vi "user info.vi"(7 "枚举":enum16{"open", "write", "read", "close"}(ring), 8 "error in":errorcluster caption="错误输出", 9 "测试条件 in":T2, 10 "粉尘特性 in":T1, 11 "Test Information in":cluster{"Test Name":string, "Tester":string}) -> (0 "error out":errorcluster, 1 "测试条件":T2, 2 "粉尘特性":T1, 3 "Test Information":cluster{"Test Name":string, "Tester":string})   [LabVIEW 2011]
uses:
  <vilib>/Utility/config.llb/Write Key (String).vi
  <vilib>/Utility/config.llb/Write Key (Double).vi
  <vilib>/Utility/config.llb/Read Key (String).vi
  <vilib>/Utility/config.llb/Read Key (Double).vi
  <vilib>/Utility/config.llb/NI_LVConfig.lvlib
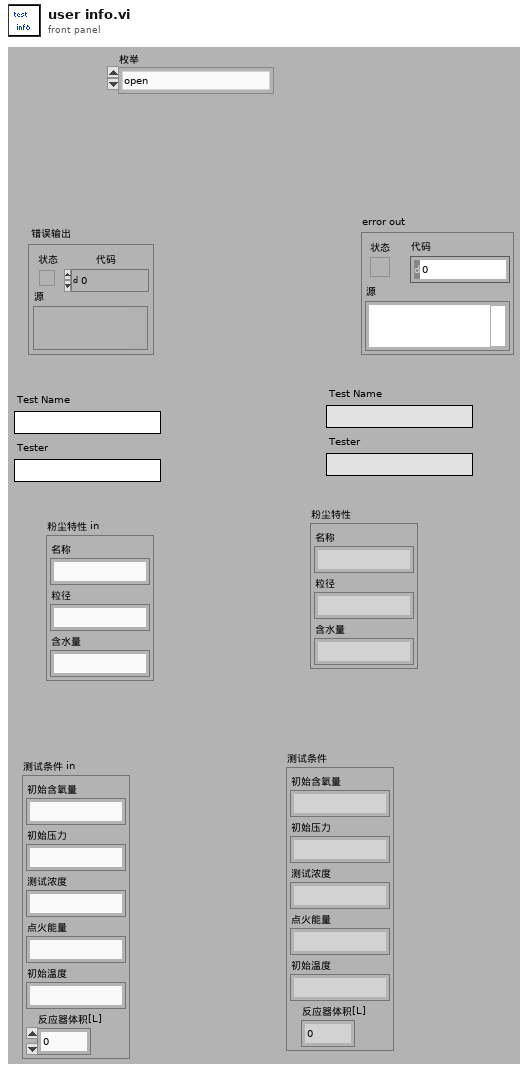
[diagram p1: front panel]
types:
  T1 = typedef "粉尘特性.ctl" = cluster{"名称":string, "粒径":string, "含水量":string}
  T2 = typedef "测试条件.ctl" = cluster{"初始含氧量":string, "初始压力":string, "测试浓度":string, "点火能量":string, "初始温度":string, "反应器体积[L]":dbl}
  T3 = typedef "NI_LVConfig.lvlib/Config Data RefNum.ctl" = refnum<k1>
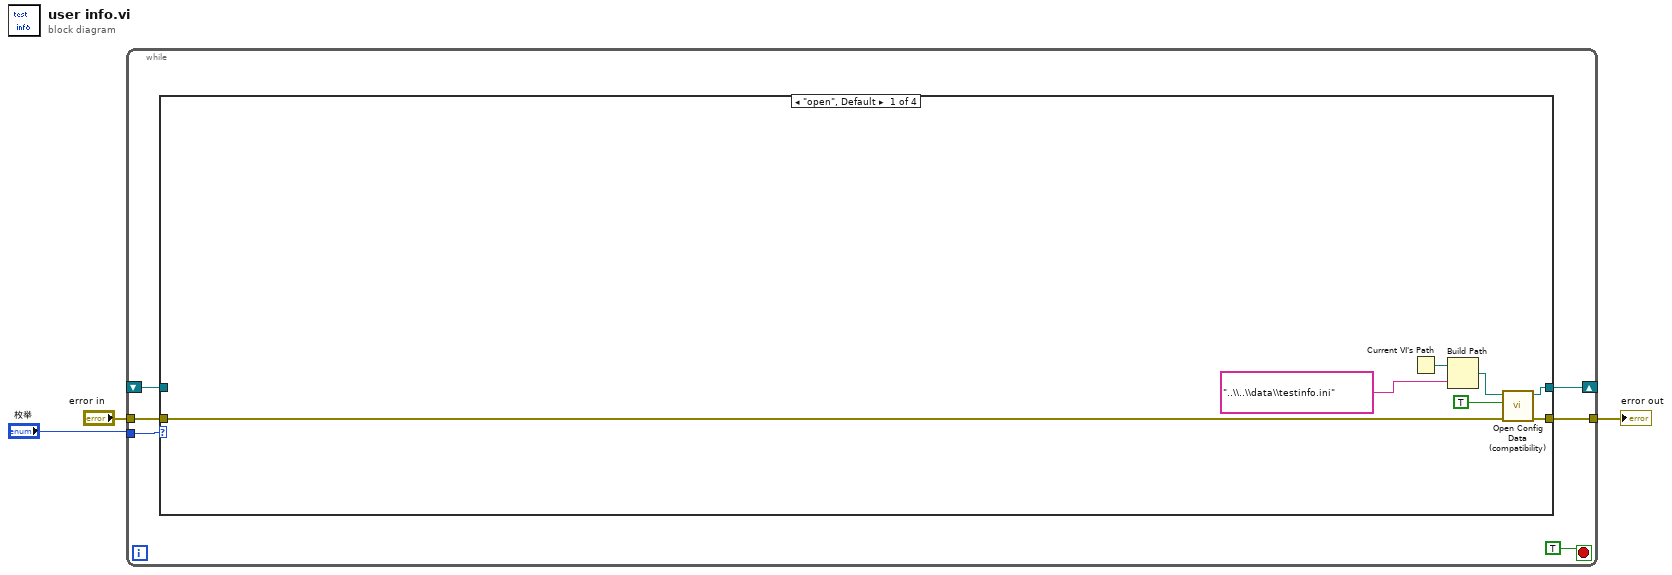
[diagram p0: block diagram]
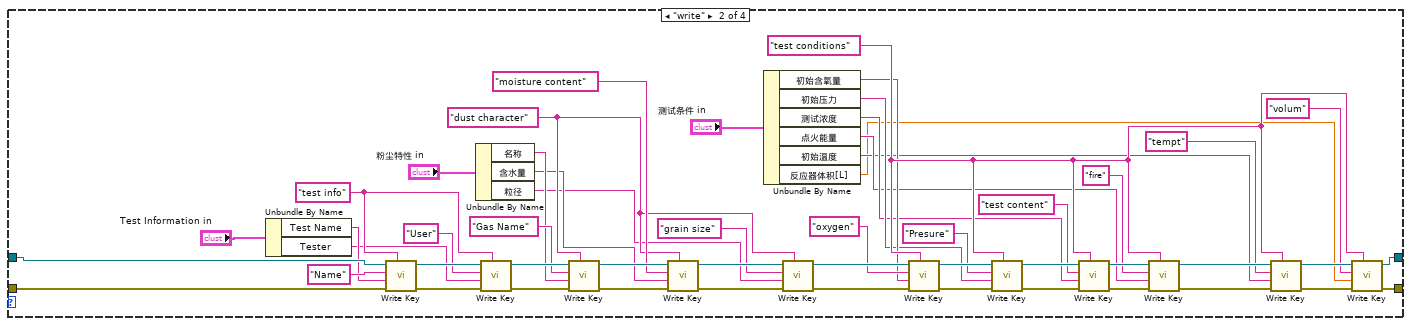
[diagram p2: hidden frame]
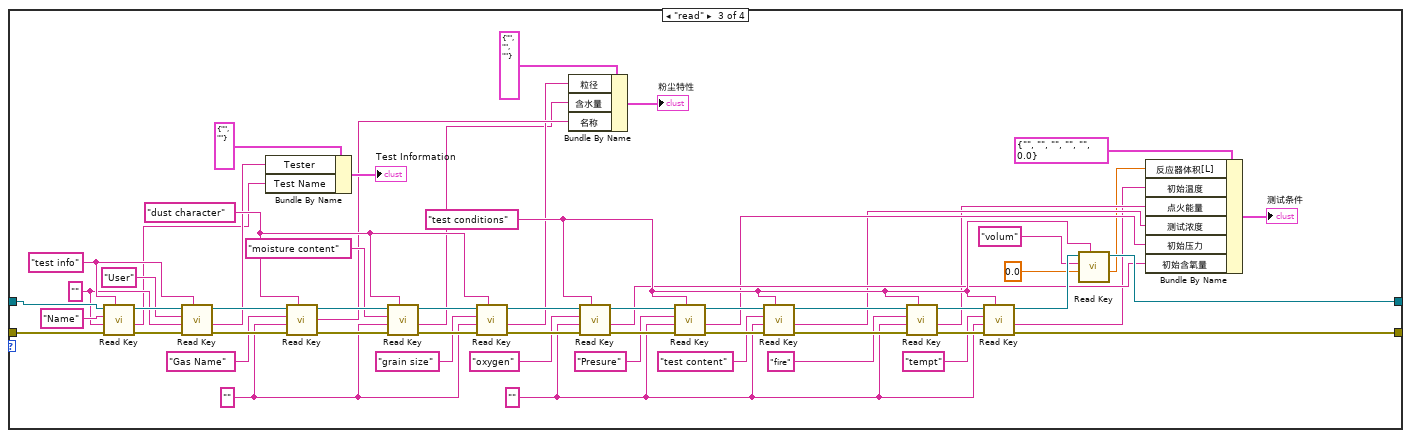
[diagram p3: hidden frame]
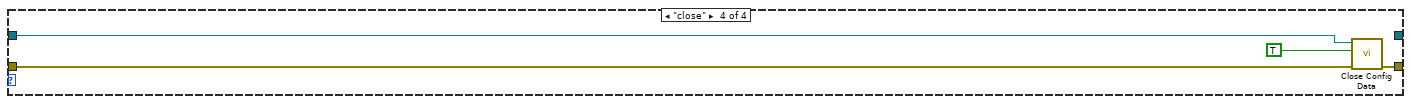
[diagram p4: hidden frame]
diagram:
  n1 = while {
    tunnel: "枚举" -> [w9]
    shift-right: [w7] -> _
    shift-left: _ -> [w6]
    tunnel: [w5] -> w1
    tunnel: "error in" -> [w4]
    stop <- TRUE stop-if-true
    n2 = case shown="\"open\", Default" w9 {
      tunnel: [w16 w34 w93 _] -> w7
      tunnel: w6 -> [_ w68 w107 w130]
      tunnel: [w15 w35 w108 w127] -> w5
      tunnel: w4 -> [w14 w55 w106 w129]
      frame "open", Default {
        n3 = Current VI's Path() -> (path=w12:path)
        n4 = Build Path(base path=w12, name or relative path="..\\..\\data\\testinfo.ini" ("名称或相对路径")) -> (appended path=w11:path)
        n5 = call <vilib>:"Open Config Data (compatibility).vi"("error in (no error)"=w14, "create file if necessary (T)"=TRUE ("create file if necessary? (T)"), "configuration file path"=w11) -> ("error out"=w15:errorcluster, "refnum"=w16:T3)  [unwired: 6 in, 1 out]
      }
      frame "write" {
        w32 = "test conditions" ("key")
        w41 = "dust character" ("key")
        w48 = "test info" ("section")
        n6 = Unbundle By Name("Test Information in") -> ("Test Name"=w29:string, "Tester"=w28:string)
        n7 = call-poly <vilib>:"Write Key.vi"("section"=w48, "error in (no error)"=w55, "value"=w29, "key"="Name", "refnum"=w68) -> ("error out"=w54:errorcluster, "refnum out"=w49:T3)  [unwired: 1 in, 4 out]
        n8 = Unbundle By Name("粉尘特性 in") -> ("名称"=w26:string, "含水量"=w25:string, "粒径"=w24:string)
        n9 = call-poly <vilib>:"Write Key.vi"("section"=w48, "error in (no error)"=w54, "value"=w28, "key"="User", "refnum"=w49) -> ("error out"=w67:errorcluster, "refnum out"=w66:T3)  [unwired: 1 in, 4 out]
        n10 = call-poly <vilib>:"Write Key.vi"("section"=w41, "error in (no error)"=w67, "value"=w26, "key"="Gas Name", "refnum"=w66) -> ("error out"=w65:errorcluster, "refnum out"=w64:T3)  [unwired: 1 in, 4 out]
        n11 = call-poly <vilib>:"Write Key.vi"("section"=w41, "error in (no error)"=w65, "value"=w25, "key"="moisture content", "refnum"=w64) -> ("error out"=w53:errorcluster, "refnum out"=w63:T3)  [unwired: 1 in, 4 out]
        n12 = Unbundle By Name("测试条件 in") -> ("初始含氧量"=w22:string, "初始压力"=w21:string, "测试浓度"=w20:string, "点火能量"=w19:string, "初始温度"=w18:string, "反应器体积[L]"=w17:dbl)
        n13 = call-poly <vilib>:"Write Key.vi"("section"=w41, "error in (no error)"=w53, "value"=w24, "key"="grain size", "refnum"=w63) -> ("error out"=w52:errorcluster, "refnum out"=w62:T3)  [unwired: 1 in, 4 out]
        n14 = call-poly <vilib>:"Write Key.vi"("section"=w32, "error in (no error)"=w52, "value"=w22, "key"="oxygen", "refnum"=w62) -> ("error out"=w51:errorcluster, "refnum out"=w61:T3)  [unwired: 1 in, 4 out]
        n15 = call-poly <vilib>:"Write Key.vi"("section"=w32, "error in (no error)"=w51, "value"=w21, "key"="Presure", "refnum"=w61) -> ("error out"=w50:errorcluster, "refnum out"=w60:T3)  [unwired: 1 in, 4 out]
        n16 = call-poly <vilib>:"Write Key.vi"("section"=w32, "error in (no error)"=w50, "value"=w20, "key"="test content", "refnum"=w60) -> ("error out"=w56:errorcluster, "refnum out"=w59:T3)  [unwired: 1 in, 4 out]
        n17 = call-poly <vilib>:"Write Key.vi"("section"=w32, "error in (no error)"=w56, "value"=w19, "key"="fire", "refnum"=w59) -> ("error out"=w57:errorcluster, "refnum out"=w58:T3)  [unwired: 1 in, 4 out]
        n18 = call-poly <vilib>:"Write Key.vi"("section"=w32, "error in (no error)"=w57, "value"=w18, "key"="tempt", "refnum"=w58) -> ("error out"=w36:errorcluster, "refnum out"=w33:T3)  [unwired: 1 in, 4 out]
        n19 = call-poly <vilib>:"Write Key.vi"("section"=w32, "error in (no error)"=w36, "value"=w17, "key"="volum", "refnum"=w33) -> ("error out"=w35:errorcluster, "refnum out"=w34:T3)  [unwired: 3 in, 2 out]
      }
      frame "read" {
        w72 = ""
        w83 = ""
        w87 = ""
        w95 = "test conditions" ("key")
        w102 = "dust character" ("key")
        w105 = "test info" ("section")
        n20 = call-poly <vilib>:"Read Key.vi"("section"=w105, "error in (no error)"=w106, "default value"=w87, "key"="Name", "refnum"=w107) -> ("error out"=w126:errorcluster, "value"=w79:string, "refnum out"=w125:T3)  [unwired: 1 in, 3 out]
        n21 = call-poly <vilib>:"Read Key.vi"("section"=w105, "error in (no error)"=w126, "default value"=w87, "key"="User", "refnum"=w125) -> ("error out"=w124:errorcluster, "value"=w86:string, "refnum out"=w123:T3)  [unwired: 1 in, 3 out]
        n22 = Bundle By Name(cluster=cluster{"Test Name":string, "Tester":string} {"Test Name"="", "Tester"=""} ("Test Information"), "Tester"=w86, "Test Name"=w79) -> (→"Test Information":cluster{"Test Name":string, "Tester":string})
        n23 = call-poly <vilib>:"Read Key.vi"("section"=w102, "error in (no error)"=w124, "default value"=w83, "key"="Gas Name", "refnum"=w123) -> ("error out"=w122:errorcluster, "value"=w82:string, "refnum out"=w121:T3)  [unwired: 1 in, 3 out]
        n24 = call-poly <vilib>:"Read Key.vi"("section"=w102, "error in (no error)"=w122, "default value"=w83, "key"="moisture content", "refnum"=w121) -> ("error out"=w120:errorcluster, "value"=w80:string, "refnum out"=w119:T3)  [unwired: 1 in, 3 out]
        n25 = call-poly <vilib>:"Read Key.vi"("section"=w102, "error in (no error)"=w120, "default value"=w83, "key"="grain size", "refnum"=w119) -> ("error out"=w118:errorcluster, "value"=w81:string, "refnum out"=w117:T3)  [unwired: 1 in, 3 out]
        n26 = Bundle By Name(cluster=T1 {"名称"="", "粒径"="", "含水量"=""} ("粉尘特性"), "粒径"=w81, "含水量"=w80, "名称"=w82) -> (→"粉尘特性":T1)
        n27 = call-poly <vilib>:"Read Key.vi"("section"=w95, "error in (no error)"=w118, "default value"=w72, "key"="oxygen", "refnum"=w117) -> ("error out"=w116:errorcluster, "value"=w76:string, "refnum out"=w115:T3)  [unwired: 1 in, 3 out]
        n28 = call-poly <vilib>:"Read Key.vi"("section"=w95, "error in (no error)"=w116, "default value"=w72, "key"="Presure", "refnum"=w115) -> ("error out"=w114:errorcluster, "value"=w75:string, "refnum out"=w113:T3)  [unwired: 1 in, 3 out]
        n29 = call-poly <vilib>:"Read Key.vi"("section"=w95, "error in (no error)"=w114, "default value"=w72, "key"="test content", "refnum"=w113) -> ("error out"=w112:errorcluster, "value"=w74:string, "refnum out"=w111:T3)  [unwired: 1 in, 3 out]
        n30 = call-poly <vilib>:"Read Key.vi"("section"=w95, "error in (no error)"=w112, "default value"=w72, "key"="fire", "refnum"=w111) -> ("error out"=w110:errorcluster, "value"=w73:string, "refnum out"=w109:T3)  [unwired: 1 in, 3 out]
        n31 = call-poly <vilib>:"Read Key.vi"("section"=w95, "error in (no error)"=w110, "default value"=w72, "key"="tempt", "refnum"=w109) -> ("error out"=w108:errorcluster, "value"=w71:string, "refnum out"=w94:T3)  [unwired: 1 in, 3 out]
        n32 = call-poly <vilib>:"Read Key.vi"("section"=w95, "default value"=0.0, "key"="volum", "refnum"=w94) -> ("value"=w69:dbl, "refnum out"=w93:T3)  [unwired: 1 in, 5 out]
        n33 = Bundle By Name(cluster=T2 {"初始含氧量"="", "初始压力"="", "测试浓度"="", "点火能量"="", "初始温度"="", "反应器体积[L]"=0.0} ("测试条件"), "反应器体积[L]"=w69, "初始温度"=w71, "点火能量"=w73, "测试浓度"=w74, "初始压力"=w75, "初始含氧量"=w76) -> (→"测试条件":T2)
      }
      frame "close" {
        n34 = call <vilib>:"Close Config Data.vi"("error in (no error)"=w129, "write file if changed (T)"=TRUE ("write configuration file? (T)"), "refnum"=w130) -> ("error out"=w127:errorcluster)  [unwired: 8 out]
      }
    }
  }
  "error out" <- w1
